vi "CHD_DRIVE_MODULE_ACQUIRE.vi"(6 "Pass_Through_Time":dbl=-1.0 format="%33.4f", 7 "Swerve Module Inx":i32, 11 "Diff Module TypDef":T1[](array[typedef])) -> (1 "Speed_MPS":dbl, 3 "Distance_M":dbl)   [LabVIEW 2019]
uses:
  <vilib>/Rock Robotics/WPI/ThirdParty/JAS_Junk/TrajLib/Trajectory_Library.lvlib
  <vilib>/Rock Robotics/SystemInterfaces/DIO/FPGA_DIOPWMChannel.ctl
  <vilib>/Rock Robotics/WPI/PWM/WPI_PWMDeadband.ctl
  <vilib>/Rock Robotics/WPI/MotorControl/WPI_MotorControlType.ctl
  <vilib>/Rock Robotics/SystemInterfaces/DIO/FPGA_DIOChannel.ctl
  <vilib>/Rock Robotics/WPI/MotorControl/WPI_MotorControlDeviceRef.ctl
  <vilib>/Rock Robotics/SystemInterfaces/Encoder/FPGA_EncoderIdx.ctl
  <vilib>/Rock Robotics/WPI/Encoder/WPI_EncoderType.ctl
  <vilib>/Rock Robotics/SystemInterfaces/Counter/FPGA_CounterCtrSystemIndex.ctl
  <vilib>/Rock Robotics/WPI/Encoder/WPI_EncoderDevRef.ctl
  CHD_DRIVE_MODULE_TYPDEF.ctl
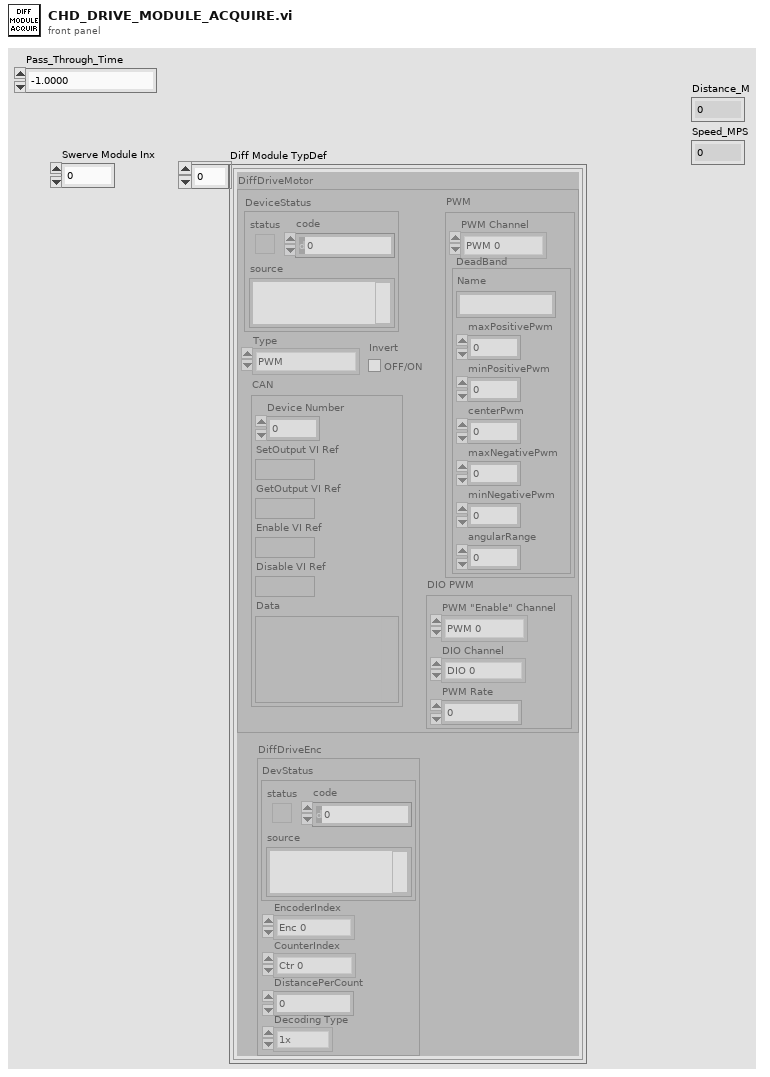
[diagram p1: front panel]
types:
  T1 = typedef "CHD_DRIVE_MODULE_TYPDEF.ctl" = cluster{"DiffDriveMotor":T2, "DiffDriveEnc":T7}
  T2 = typedef "WPI_MotorControlDeviceRef.ctl" = cluster{"DeviceStatus":errorcluster, "Type":T3, "PWM":cluster{"PWM Channel":T4, "DeadBand":T5}, "CAN":cluster{"Device Number":u8, "SetOutput VI Ref":variant, "GetOutput VI Ref":variant, "Enable VI Ref":variant, "Disable VI Ref":variant, "Data":variant}, "Invert":bool, "DIO PWM":cluster{"PWM \"Enable\" Channel":T4, "DIOChannel":T6, "PWM Rate":dbl}}
  T3 = typedef "WPI_MotorControlType.ctl" = enum16{"PWM", "CAN", "DIO PWM"}
  T4 = typedef "FPGA_DIOPWMChannel.ctl" = enum8{"PWM 0", "PWM 1", "PWM 2", "PWM 3", "PWM 4", "PWM 5", "PWM 6", "PWM 7", "PWM 8", "PWM 9", "PWM MXP 0", "PWM MXP 1", "PWM MXP 2", "PWM MXP 3", "PWM MXP 4", "PWM MXP 5", "PWM MXP 6", "PWM MXP 7", "PWM MXP 8", "PWM MXP 9", "Invalid"}
  T5 = typedef "WPI_PWMDeadband.ctl" = cluster{"Name":string, "maxPositivePwm":i32, "minPositivePwm":i32, "centerPwm":i32, "maxNegativePwm":i32, "minNegativePwm":i32, "angularRange":u16}
  T6 = typedef "FPGA_DIOChannel.ctl" = enum8{"DIO 0", "DIO 1", "DIO 2", "DIO 3", "DIO 4", "DIO 5", "DIO 6", "DIO 7", "DIO 8", "DIO 9", "DIO MXP 0", "DIO MXP 1", "DIO MXP 2", "DIO MXP 3", "DIO MXP 4", "DIO MXP 5", "DIO MXP 6", "DIO MXP 7", "DIO MXP 8", "DIO MXP 9", "DIO MXP 10", "DIO MXP 11", "DIO MXP 12", "DIO MXP 13", "DIO MXP 14", "DIO MXP 15", "SPI Port CS1", "SPI Port CS2", "SPI Port CS3", "SPI Port MISO", "SPI Port MOSI", "Invalid"}
  T7 = typedef "WPI_EncoderDevRef.ctl" = cluster{"DevStatus":errorcluster, "EncoderIndex":T8, "CounterIndex":T9, "DistancePerCount":dbl, "Decoding Type":T10}
  T8 = typedef "FPGA_EncoderIdx.ctl" = enum8{"Enc 0", "Enc 1", "Enc 2", "Enc 3", "Enc 4", "Enc 5", "Enc 6", "Enc 7", "Invalid"}
  T9 = typedef "FPGA_CounterCtrSystemIndex.ctl" = enum8{"Ctr 0", "Ctr 1", "Ctr 2", "Ctr 3", "Ctr 4", "Ctr 5", "Ctr 6", "Ctr 7", "Invalid"}
  T10 = typedef "WPI_EncoderType.ctl" = enum16{"1x", "2x", "4x"}
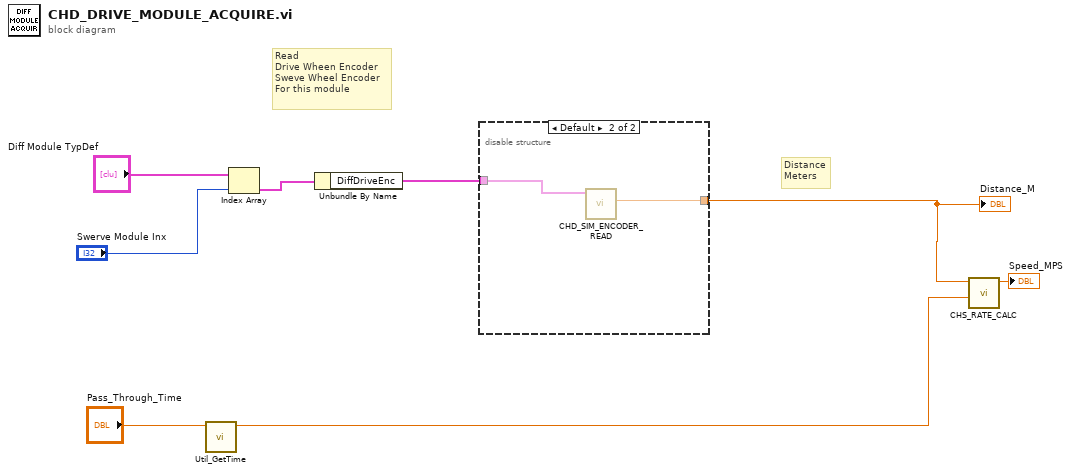
[diagram p0: block diagram]
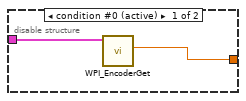
[diagram p2: hidden frame]
diagram:
  # "Read \nDrive Wheen Encoder\nSweve Wheel Encoder\nFor this module"
  # "Distance\nMeters"
  n1 = call <vilib>:"Util_GetTime.vi"("Pass_Through_Time"="Pass_Through_Time") -> ("FPGA_Time_Seconds"=w7:dbl)  [unwired: 8 in, 2 out]
  n2 = Index Array(array="Diff Module TypDef", index="Swerve Module Inx") -> (element=w4:T1)
  n3 = Unbundle By Name(w4) -> ("DiffDriveEnc"=w3:T7)
  n4 = disable-structure shown="Default" {
    disable-tunnel: w3 -> [w10 w12]
    disable-tunnel: [w9 w11] -> w2
    frame condition #0 (active) {
      n5 = call <vilib>:"WPI_EncoderGet.vi"("EncoderDevRef"=w10) -> ("Distance"=w9:dbl)  [unwired: 5 in, 5 out]
    }
    frame condition #1 {
      n6 = call "CHD_SIM_ENCODER_READ.vi"("EncoderReference"=w12) -> ("Distance"=w11:dbl)  [unwired: 9 in, 1 out]
    }
  }
  "Distance_M" <- w2
  n7 = call "CHS_RATE_CALC.vi"("Time"=w7, "Input"=w2) -> ("Output"=→"Speed_MPS":dbl)  [unwired: 9 in]
